vi "add_WrenchStamped.vi"(5 "Wrench":T1, 6 "Stamp":cluster{"frame_id":string, "reset seq?":bool}, 7 "msg in":string) -> (3 "msg out":string)   [LabVIEW 2012]
doc: "Flattens a wrench stamped into a message"
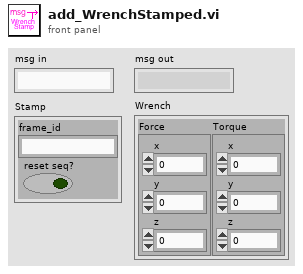
[diagram p1: front panel]
types:
  T1 = cluster{"Force":cluster{"x":dbl, "y":dbl, "z":dbl}, "Torque":cluster{"x":dbl, "y":dbl, "z":dbl}}
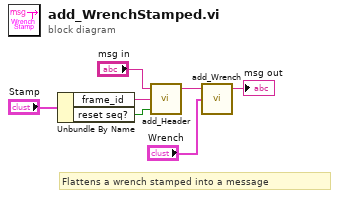
[diagram p0: block diagram]
diagram:
  # "Flattens a wrench stamped into a message"
  n1 = Unbundle By Name("Stamp") -> ("frame_id"=w2:string, "reset seq?"=w1:bool)
  n2 = call <userlib>:"add_Header.vi"("reset seq?"=w1, "frame_id"=w2, "msg in"="msg in") -> ("msg out"=w6:string)  [unwired: 2 in]
  n3 = call "add_Wrench.vi"("Wrench"="Wrench", "msg in"=w6) -> ("msg out"=→"msg out":string)  [unwired: 3 in]
